vi "Get FXP VI Ref.vi"(7 "Channel Type":T1, 8 "error in (no error)":errorcluster, 11 "FXP Config in":T2) -> (0 "error out":errorcluster, 2 "FXP VI Ref":refnum<vi>, 3 "FXP Config out":T2)   [LabVIEW 2011, in "Scan Engine Custom Device.lvlib"]
uses:
  Scan Engine Custom Device.lvlib
  Type Defs/FXP Config.ctl
  <vilib>/NI Veristand/Custom Device API/Custom Device Channel Type.ctl
  Globals/String Constants.vi
  <vilib>/NI Veristand/Custom Device API/Custom Device API.lvlib
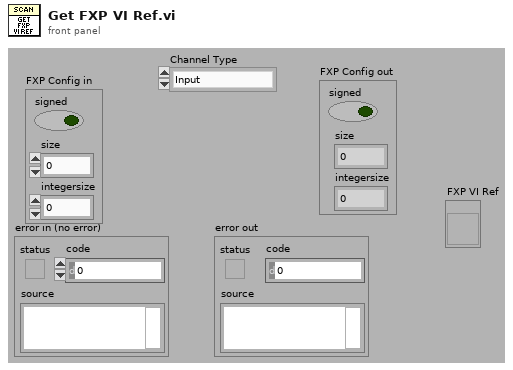
[diagram p1: front panel]
types:
  T1 = typedef "Custom Device API.lvlib/Custom Device Channel Type.ctl" = enum16{"Input", "Output"}
  T2 = typedef "Scan Engine Custom Device.lvlib/FXP Config.ctl" = cluster{"signed":bool, "size":u32, "integersize":i32}
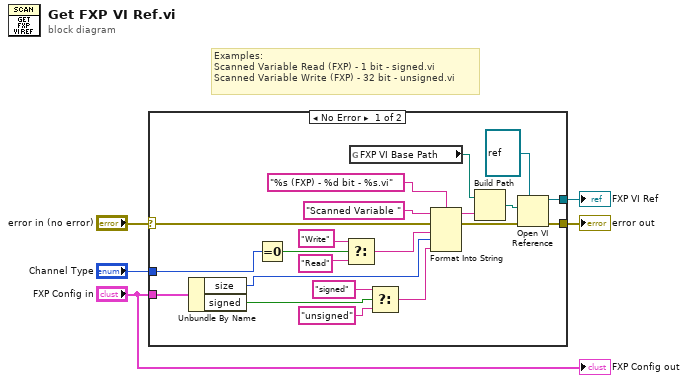
[diagram p0: block diagram]
diagram:
  # "Examples:\nScanned Variable Read (FXP) - 1 bit - signed.vi\nScanned Variable Write (FXP) - 32 bit - unsigned.vi"
  n1 = case shown="No Error" "error in (no error)" {
    selector: "error in (no error)" -> [w17 w27]
    tunnel: [w26 w27] -> w5
    tunnel: [w25 _] -> w1
    tunnel: "FXP Config in" -> [w24 _]
    tunnel: "Channel Type" -> [w11 _]
    frame No Error {
      n2 = Unbundle By Name(w24) -> ("size"=w12:u32, "signed"=w20:bool)
      n3 = Equal To 0?(x=w11) -> (x = 0?=w10:bool)
      n4 = Select(t="Write" ("initial string"), s=w10, f="Read" ("initial string")) -> (s? t:f=w7:string)
      n5 = global read "String Constants.vi" "FXP VI Base Path"() -> (w23:path)
      n6 = Select(t="signed" ("initial string"), s=w20, f="unsigned" ("initial string")) -> (s? t:f=w13:string)
      n7 = Format Into String(format string="%s (FXP) - %d bit - %s.vi", initial string="Scanned Variable ", error in=w17, w7, w12, w13) -> (resulting string=w15:string, error out=w16:errorcluster)
      n8 = Build Path(base path=w23, name or relative path=w15) -> (appended path=w14:path)
      n9 = Open VI Reference(type specifier VI Refnum (for type only)=refnum<vi> refnum ("FXP VI Ref"), vi path=w14, error in (no error)=w16) -> (vi reference=w25:refnum<vi>, error out=w26:errorcluster)  [unwired: 3 in]
    }
    frame Error {
    }
  }
  "error out" <- w5
  "FXP VI Ref" <- w1
  "FXP Config out" <- "FXP Config in"
